vi "Vision Processing.vi"(4 "error in (no error)":errorcluster, 5 "Camera Type":enum16{"206", "1011"}(ring)=enum."1011") -> ()   [LabVIEW 2011]
uses:
  Robot Global Data.vi
  <vilib>/vision/NI_Vision_Development_Module.lvlib
panel:
  in  "View":bool=TRUE
  out "Target Info":T1(array[cluster])
  in  "Area Size Limit":i32=444
  in  "Particle Count Limit":i32=4
  in  "Score Limits":T2={"Rect Coverage"=76.0, "Aspect Ratio"=70.0, "X Edge Strength"=40.0, "Y Edge Strength"=60.0}
  in  "Processing":enum32{"Color", "Intensity", "Intensity Open"}(tab)
  in  "Luminance":i32=150
  in  "Saturation":i32=120
  in  "Hue":i32(knob)=100 scale=0.0..255.0
  in  "Margins":cluster{"Hue":i32, "Sat":i32, "Lum":i32}={"Hue"=20, "Sat"=40, "Lum"=40} {"Sat" scale=0.0..40.0; "Lum" scale=0.0..40.0; "Hue" scale=0.0..40.0}
  in  "Range":cluster{"Lower value":sgl, "Upper value":sgl}={"Lower value"=150.0, "Upper value"=255.0} {"Lower value" scale=0.0..255.0; "Upper value" scale=0.0..255.0}
  in  "Range":cluster{"Lower value":sgl, "Upper value":sgl}={"Lower value"=150.0, "Upper value"=255.0} {"Lower value" scale=0.0..255.0; "Upper value" scale=0.0..255.0}
  in  "View":bool=TRUE
  out "Processed Image":T3(plugin-control)
  out "Original Image":T3(plugin-control)
  # "Instructions:\nProcessing the reflective tape that is illuminated by a ring light can be based\non color or light intensity.\nParticles within the image are scored by rectangle coverage, aspect ratio, and\nfor being hollow with a bold edge. A particle is considered a target if all scores\nare above the score limits. Particles can be annotated -- surrounded by\na rectangle and scores drawn to the left .\nTo control the number of particles being scored, use the count limit and the size\nlimit."
  # "To debug, Enable using the View button.\nFor color processing, you can click in the image to select the color for processing."
  # "Enable by clicking the View button.\nGreen scores are above the limit, orange are below. Inner/outer rect\nindicates all passed."
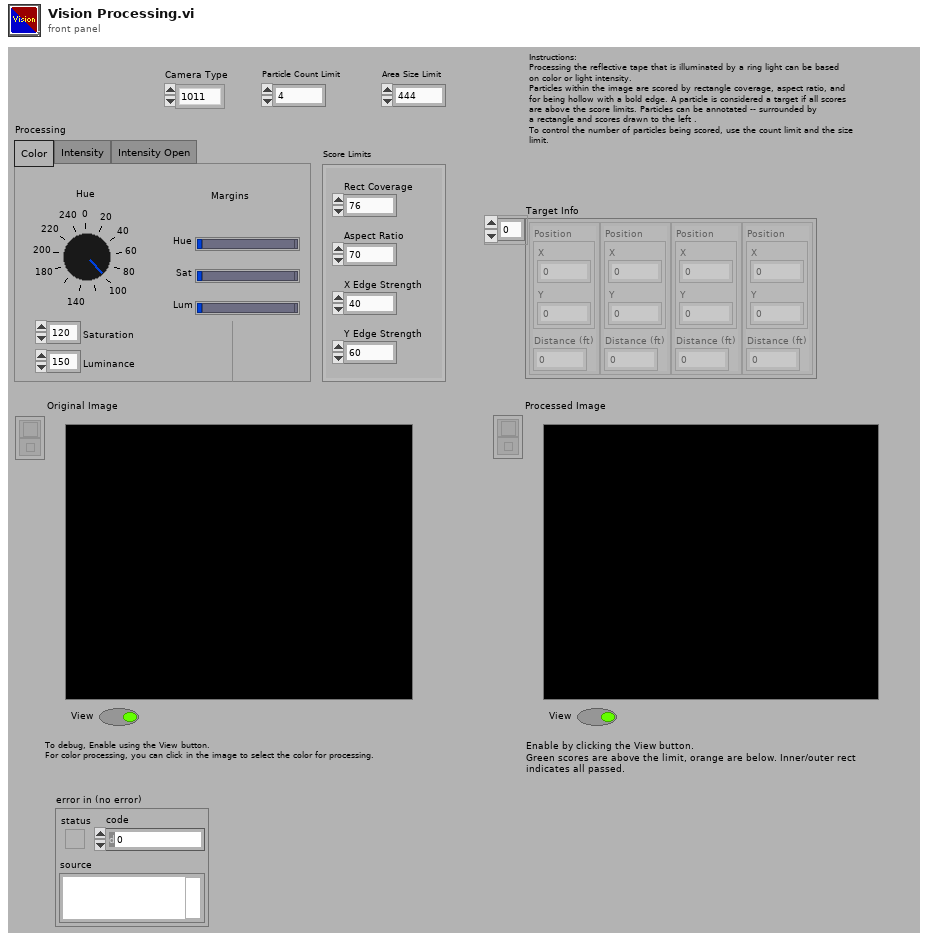
[diagram p1: front panel]
types:
  T1 = cluster{"Position":cluster{"X":dbl, "Y":dbl}, "Distance (ft)":dbl}[]
  T2 = cluster{"Rect Coverage":dbl, "Aspect Ratio":dbl, "X Edge Strength":dbl, "Y Edge Strength":dbl}
  T3 = typedef "IMAQ Image.ctl" = refnum<image>
  T4 = typedef "WPI_DriverStationRobotMode.ctl" = enum16{"Autonomous Disabled", "Autonomous Enabled", "Teleop Disabled", "Teleop Enabled", "Timeout", "Finish"}
  T5 = enum32{"AutoM", "Close", "Dilate", "Erode", "Gradient", "Gradient out", "Gradient in", "Hit miss", "Open", "PClose", "POpen", "Thick", "Thin"}
  T6 = typedef "Image Type" = u32
  T7 = typedef "WPI_CameraDevRef.ctl" = cluster{"Camera Address":string, "CameraStatus":errorcluster, "Acquire Image Notifier":refnum<notifier>}
  T8 = cluster{"Activate Elevator":bool, "Shoot":bool, "Bridge Direction":bool, "Low Speed":bool, "Med Speed":bool, "High Speed":bool, "Loader Down":bool, "Activate Bridge":bool, "Limit Shooter":bool, "Elevator Down":bool, "Reverse":bool, "Vision Processing":bool}
  T9 = typedef "WPI_CameraImageSize.ctl" = enum16{"640x480", "320x240", "160x120"}
  T10 = cluster{cluster{"Left":dbl, "Top":dbl, "Right":dbl, "Bottom":dbl}, dbl[]}[]
  T11 = cluster{"Left":dbl, "Top":dbl, "Right":dbl, "Bottom":dbl}
  T12 = cluster{"Target Center (-1 to 1)":cluster{"X":dbl, "Y":dbl}, "Distance (ft)":dbl}
  T13 = cluster{"Target Center (-1 to 1)":cluster{"X":dbl, "Y":dbl}, "Distance (ft)":dbl}[]
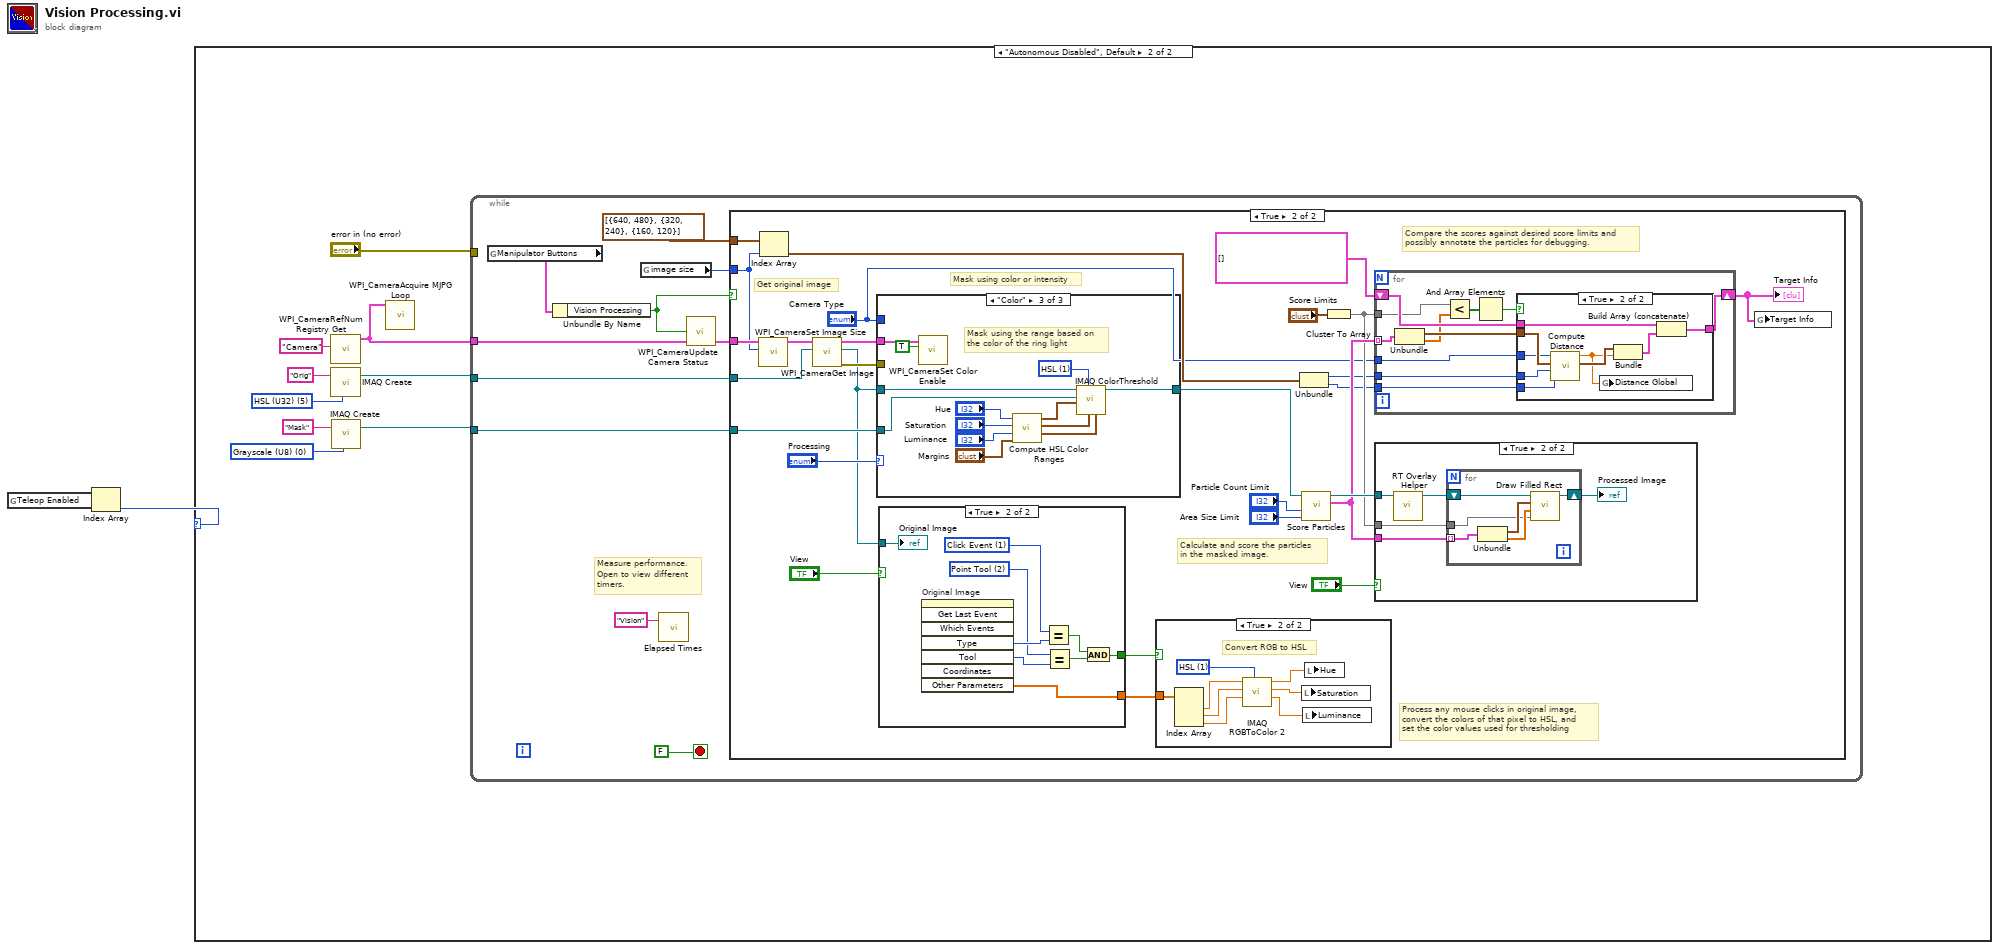
[diagram p0: block diagram]
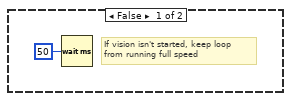
[diagram p3: hidden frame]
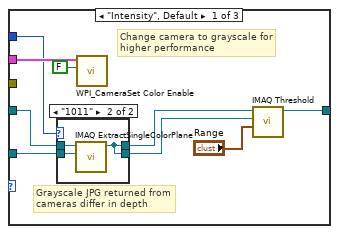
[diagram p5: hidden frame]
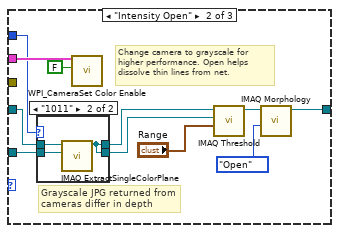
[diagram p7: hidden frame]
diagram:
  n1 = global read "Robot Global Data.vi" "Teleop Enabled"() -> (w2:T4[])
  n2 = Index Array(array=w2) -> (element=w1:T4)  [unwired: 1 in]
  n3 = case shown="\"Autonomous Disabled\", Default" w1 {
    frame "Autonomous Enabled" {
    }
    frame "Autonomous Disabled", Default {
      w6 = T6 0 items=["Grayscale (U8)", "Grayscale (I16)", "Grayscale (SGL)", "Complex (CSG)", "RGB (U32)", "HSL (U32)", "RGB (U64)", "Grayscale (U16)"] ("Image Type")
      w10 = T6 5 items=["Grayscale (U8)", "Grayscale (I16)", "Grayscale (SGL)", "Complex (CSG)", "RGB (U32)", "HSL (U32)", "RGB (U64)", "Grayscale (U16)"] ("Image Type")
      n4 = call <vilib>:"WPI_CameraRefNum Registry Get.vi"("refnum name"="Camera") -> ("CameraDevRef"=w8:T7)  [unwired: 9 in, 1 out]
      n5 = call "IMAQ Create"("Image Name"="Orig", "Image Type"=w10) -> ("New Image"=w9:T3)  [unwired: 2 in, 2 out]
      n6 = call "IMAQ Create"("Image Name"="Mask", "Image Type"=w6) -> ("New Image"=w4:T3)  [unwired: 2 in, 2 out]
      n7 = call <vilib>:"WPI_CameraAcquire MJPG Loop.vi"("CameraDevRef"=w8) -> ()  [unwired: 11 in]
      n8 = while {
        tunnel: w9 -> [w20]
        tunnel: w8 -> [w19]
        tunnel: "error in (no error)" -> [_]
        tunnel: w4 -> [w15]
        stop <- FALSE stop-if-true
        # "Measure performance.\nOpen to view different\ntimers."
        n9 = global read "Robot Global Data.vi" "Manipulator Buttons"() -> (w13:T8)
        n10 = Unbundle By Name(w13) -> ("Vision Processing"=w12:bool)
        n11 = global read "Robot Global Data.vi" "image size"() -> (w16:T9)
        n12 = call "Elapsed Times.vi"("Call Name"="Vision") -> ()  [unwired: 2 in, 1 out]
        n13 = call <vilib>:"WPI_CameraUpdate Camera Status.vi"("CameraDevRef In"=w19, "Enable Vision"=w12) -> ("CameraDevRef Out"=w18:T7)  [unwired: 3 in]
        n14 = case shown="True" w12 {
          tunnel: w20 -> [_ w40]
          tunnel: w18 -> [_ w35]
          tunnel: w16 -> [_ w30]
          tunnel: w15 -> [_ w25]
          tunnel: cluster{i32, i32}[] [{640, 480}, {320, 240}, {160, 120}] -> [_ w29]
          frame False {
            # "If vision isn't started, keep loop\nfrom running full speed"
            n15 = Wait (ms)(milliseconds to wait=u32 50) -> ()  [unwired: 1 out]
          }
          frame True {
            # "Compare the scores against desired score limits and\npossibly annotate the particles for debugging."
            # "Process any mouse clicks in original image,\nconvert the colors of that pixel to HSL, and\nset the color values used for thresholding"
            # "Calculate and score the particles\nin the masked image."
            # "Mask using color or intensity"
            # "Get original image"
            n16 = call <vilib>:"WPI_CameraSet Image Size.vi"("Image Size"=w30, "CameraDevRef"=w35) -> ("CameraDevRef Out"=w36:T7)  [unwired: 8 in, 1 out]
            n17 = Index Array(array=w29, index=w30) -> (element=w26:cluster{i32, i32})
            n18 = call <vilib>:"WPI_CameraGet Image.vi"("Image"=w40, "CameraDevRef"=w36) -> ("error out"=w38:errorcluster, "Image Out"=w24:T3, "CameraDevRef Out"=w39:T7)  [unwired: 7 in]
            n19 = case shown="\"Color\"" "Processing" {
              tunnel: w24 -> [w62 w74 w100]
              tunnel: [w65 w79 w99] -> w33
              tunnel: w39 -> [w63 w77 w90]
              tunnel: w38 -> [_ _ _]
              tunnel: w25 -> [w61 w75 w88]
              tunnel: "Camera Type" -> [w60 w76 _]
              frame "Intensity", Default {
                # "Grayscale JPG returned from\ncameras differ in depth"
                # "Change camera to grayscale for\nhigher performance"
                n20 = case shown="\"1011\"" w60 {
                  tunnel: w62 -> [w68 w71]
                  tunnel: w61 -> [w67 w70]
                  tunnel: [w68 w69] -> w59
                  tunnel: [w67 w69] -> w58
                  frame "206", Default {
                  }
                  frame "1011" {
                    n21 = call "IMAQ ExtractSingleColorPlane"("Image Dst"=w70, "Image Src"=w71) -> ("Image Dst Out"=w69:T3)  [unwired: 8 in, 1 out]
                  }
                }
                n22 = call <vilib>:"WPI_CameraSet Color Enable.vi"("Color Enabled"=FALSE, "CameraDevRef"=w63) -> ()  [unwired: 8 in, 2 out]
                n23 = call "IMAQ Threshold"("Range"="Range", "Image Dst"=w58, "Image Src"=w59) -> ("Image Dst Out"=w65:T3)  [unwired: 3 in, 5 out]
              }
              frame "Intensity Open" {
                # "Grayscale JPG returned from\ncameras differ in depth"
                # "Change camera to grayscale for\nhigher performance. Open helps\ndissolve thin lines from net."
                n24 = case shown="\"1011\"" w76 {
                  tunnel: w74 -> [w84 w87]
                  tunnel: w75 -> [w83 w86]
                  tunnel: [w84 w85] -> w73
                  tunnel: [w83 w85] -> w72
                  frame "206", Default {
                  }
                  frame "1011" {
                    n25 = call "IMAQ ExtractSingleColorPlane"("Image Dst"=w86, "Image Src"=w87) -> ("Image Dst Out"=w85:T3)  [unwired: 8 in, 1 out]
                  }
                }
                n26 = call <vilib>:"WPI_CameraSet Color Enable.vi"("Color Enabled"=FALSE, "CameraDevRef"=w77) -> ()  [unwired: 8 in, 2 out]
                n27 = call "IMAQ Threshold"("Range"="Range", "Image Dst"=w72, "Image Src"=w73) -> ("Image Dst Out"=w80:T3)  [unwired: 3 in, 5 out]
                n28 = call "IMAQ Morphology"("Operation"=T5."Open", "Image Src"=w80) -> ("Image Dst Out"=w79:T3)  [unwired: 8 in, 1 out]
              }
              frame "Color" {
                w98 = u16 1 items=["RGB", "HSL", "HSV", "HSI"] ("Color Mode")
                # "Mask using the range based on\nthe color of the ring light"
                n29 = call <vilib>:"WPI_CameraSet Color Enable.vi"("Color Enabled"=TRUE, "CameraDevRef"=w90) -> ()  [unwired: 8 in, 2 out]
                n30 = call "Compute HSL Color Ranges.vi"("Margins"="Margins", "Luminance"="Luminance", "Saturation"="Saturation", "Hue"="Hue") -> ("Lum Range"=w95:cluster{i32, i32}, "Sat Range"=w96:cluster{i32, i32}, "Hue Range"=w97:cluster{i32, i32})  [unwired: 5 in]
                n31 = call "IMAQ ColorThreshold"("Blue or Luma or Val or Inten Range"=w95, "Green or Sat Range"=w96, "Color Mode"=w98, "Red or Hue Range"=w97, "Image Dst"=w88, "Image Src"=w100) -> ("Image Dst Out"=w99:T3)  [unwired: 4 in, 1 out]
              }
            }
            n32 = case shown="True" "View" {
              tunnel: w24 -> [_ w120]
              tunnel: [_ w115] -> w32
              tunnel: [_ w112] -> w31
              frame False {
              }
              frame True {
                w113 = 2 items=["None", "Selection Tool", "Point Tool", "Line Tool", "Rectangle Tool", "Oval Tool", "Polygon Tool", "ClosedFreehandTool", "Annulus Tool", "Rotated Rectangle Tool", "Zoom Tool", "Pan Tool", "Polyline Tool", "Freehand Tool"] ("Tool")
                w114 = 1 items=["No Event"=0, "Click Event"=1, "Draw Event"=2, "Size Event"=4, "Scroll Event"=5, "Double Click Event"=8] ("Type")
                n33 = invoke on="Original Image" class="ImageControl" method="Get Last Event"() -> ("Type"=w116:i32, "Tool"=w119:i32, "Other Parameters"=w112:sgl[])  [unwired: 8 in, 5 out]
                n34 = Equal?(x=w114, y=w116) -> (x = y?=w117:bool)
                n35 = Equal?(x=w113, y=w119) -> (x = y?=w118:bool)
                n36 = And(x=w117, y=w118) -> (x .and. y?=w115:bool)
                "Original Image" <- w120
              }
            }
            n37 = case shown="True" w32 {
              tunnel: w31 -> [_ w57]
              frame False {
              }
              frame True {
                w56 = u16 1 items=["RGB", "HSL", "HSV", "HSI", "CIE L*a*b*", "CIE XYZ"] ("Color Mode")
                # "Convert RGB to HSL"
                n38 = Index Array(array=w57) -> (element #1=w55:sgl, element #2=w53:sgl, element #3=w51:sgl)  [unwired: 3 in]
                n39 = call "IMAQ RGBToColor 2"("Color Mode"=w56, "Blue value"=w51, "Green value"=w53, "Red value"=w55) -> ("Blue or Luma or Val or Inten or Z or b*value"=w50:dbl, "Green or Sat or Y or a* value"=w52:dbl, "Red or Hue or X or L* value"=w54:dbl)  [unwired: 4 in, 1 out]
                n40 = local write "Saturation"(w52) -> ()
                n41 = local write "Luminance"(w50) -> ()
                n42 = local write "Hue"(w54) -> ()
              }
            }
            n43 = Unbundle(w26) -> (w28:i32, w27:i32)
            n44 = call "Score Particles.vi"("Area Size Limit"="Area Size Limit", "Particle Count Limit"="Particle Count Limit", "Image Refnum in"=w33) -> ("Scored Particle Info"=w45:T10, "Image Refnum out"=w48:T3)  [unwired: 7 in]
            n45 = Cluster To Array(cluster="Score Limits") -> (array=w43:dbl[])
            n46 = for {
              shift-right: [w130] -> w37
              shift-left: T1 [] -> [w131]
              tunnel: w28 -> [w129]
              tunnel: w45 -> [w127] mode=indexing
              tunnel: w43 -> [w122]
              tunnel: "Camera Type" -> [w126]
              tunnel: w27 -> [w121]
              n47 = Unbundle(w127) -> (w128:T11, w123:dbl[])
              n48 = Less?(x=w122, y=w123) -> (x < y?=w125:bool[])
              n49 = And Array Elements(Boolean array=w125) -> (logical AND=w124:bool)
              n50 = case shown="True" w124 {
                tunnel: w131 -> [w132 w141]
                tunnel: [w132 w140] -> w130
                tunnel: w128 -> [_ w137]
                tunnel: w129 -> [_ w138]
                tunnel: w126 -> [_ w136]
                tunnel: w121 -> [_ w135]
                frame False {
                }
                frame True {
                  n51 = call "Compute Distance.vi"("Y Image Resolution"=w135, "X Image Resolution"=w138, "Bounding Box"=w137, "Camera Type"=w136) -> ("Target Center (-1 to 1)"=w134:cluster{"X":dbl, "Y":dbl}, "Distance (ft)"=w133:dbl)  [unwired: 6 in]
                  n52 = global write "Robot Global Data.vi" "Distance Global"(w133) -> ()
                  n53 = Bundle("Target Center (-1 to 1)"=w134, "Distance (ft)"=w133) -> (w139:T12)  [unwired: 1 in]
                  n54 = Build Array (concatenate) "Build Array"(w141, w139) -> (w140:T13)
                }
              }
            }
            "Target Info" <- w37
            n55 = case shown="True" "View" {
              tunnel: w48 -> [_ w102]
              tunnel: w45 -> [_ w104]
              tunnel: w43 -> [_ w103]
              frame False {
              }
              frame True {
                n56 = call "RT Overlay Helper.vi"("Refnum in"=w102) -> ("Refnum out"=w105:T3)  [unwired: 10 in]
                n57 = for {
                  shift-right: [w110] -> w101
                  shift-left: w105 -> [w111]
                  tunnel: w104 -> [w107] mode=indexing
                  tunnel: w103 -> [w106]
                  n58 = Unbundle(w107) -> (w108:T11, w109:dbl[])
                  n59 = call "Draw Filled Rect.vi"("Limits"=w106, "Scores"=w109, "Bounding Box"=w108, "image in"=w111) -> ("image out"=w110:T3)  [unwired: 7 in]
                }
                "Processed Image" <- w101
              }
            }
            n60 = global write "Robot Global Data.vi" "Target Info"(w37) -> ()
          }
        }
      }
    }
  }
